vi "Clase3.vi"() -> ()   [LabVIEW 2011]
panel:
  out "Alarma":string
  out "Observación":string
  out "Alarma":bool
  out "Velocidad":i32(knob) scale=1.0..180.0
  out "Temperatura":dbl(slide) scale=0.0..100.0
  # "Generar la temperatura entre 1-100 y la velocidad entre 1-180 cuando la velocidad sea mayor a 100 debemos de\nescribir velocidad ALTA y cuando la temperatura sea mayor a 80 y la velocidad mayor a 120, se debe de encender \nla alarma."
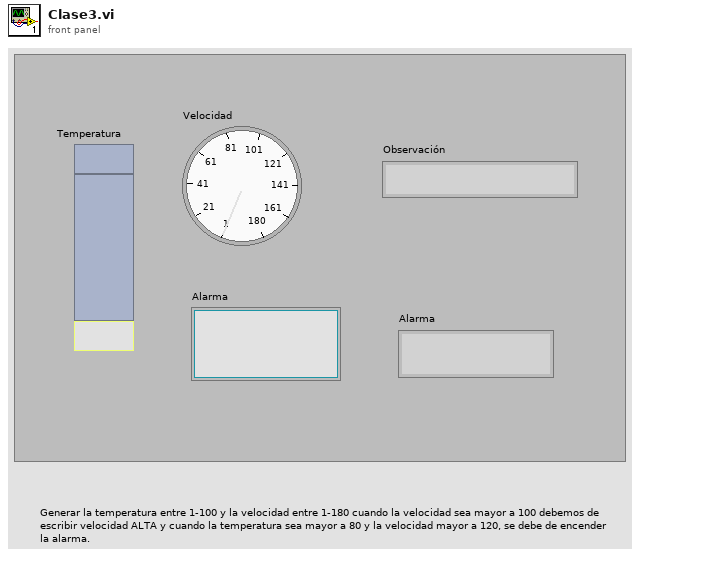
[diagram p1: front panel]
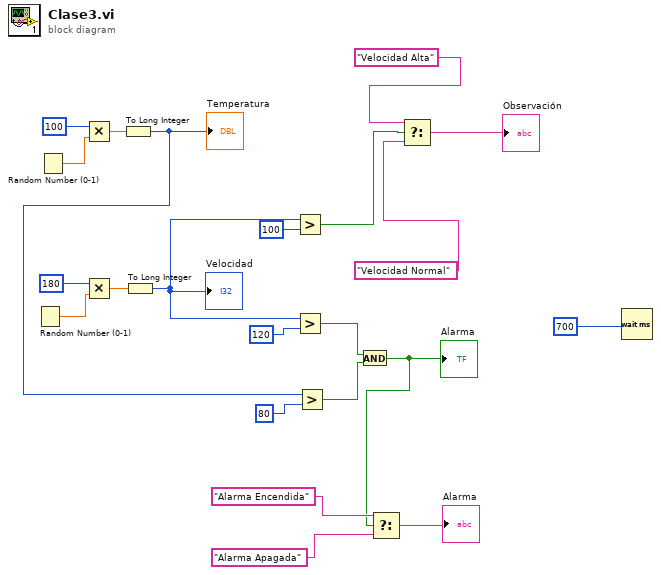
[diagram p0: block diagram]
diagram:
  n1 = Random Number (0-1)() -> (number: 0 to 1=w21:dbl)
  n2 = Random Number (0-1)() -> (number: 0 to 1=w19:dbl)
  n3 = Multiply(x=100, y=w19) -> (x*y=w17:dbl)
  n4 = Multiply(x=180, y=w21) -> (x*y=w18:dbl)
  n5 = To Long Integer(number=w17) -> (32bit integer=w9:i32)
  "Temperatura" <- w9
  n6 = To Long Integer(number=w18) -> (32bit integer=w11:i32)
  "Velocidad" <- w11
  n7 = Greater?(x=w11, y=100) -> (0:w14:bool)
  n8 = Greater?(x=w11, y=120) -> (0:w7:bool)
  n9 = Greater?(x=w9, y=80) -> (0:w6:bool)
  n10 = And(x=w7, y=w6) -> (x .and. y?=w2:bool)
  "Alarma" <- w2
  n11 = Select(t="Alarma Encendida", s=w2, f="Alarma Apagada") -> (s? t:f=→"Alarma":string)
  n12 = Select(t="Velocidad Alta", s=w14, f="Velocidad Normal") -> (s? t:f=→"Observación":string)
  n13 = Wait (ms)(milliseconds to wait=700 ("y")) -> ()  [unwired: 1 out]
